vi "8_1_2.vi"() -> ()   [LabVIEW 2021, in "2022.lvlib"]
uses:
  2022.lvlib
panel:
  in  "8_1/2":bool=TRUE
  out "max value":i32
  out "size(s)":i32
  out "Array 2":bool[][](array[boolean])
  out "Array":i32[][](array[numeric])
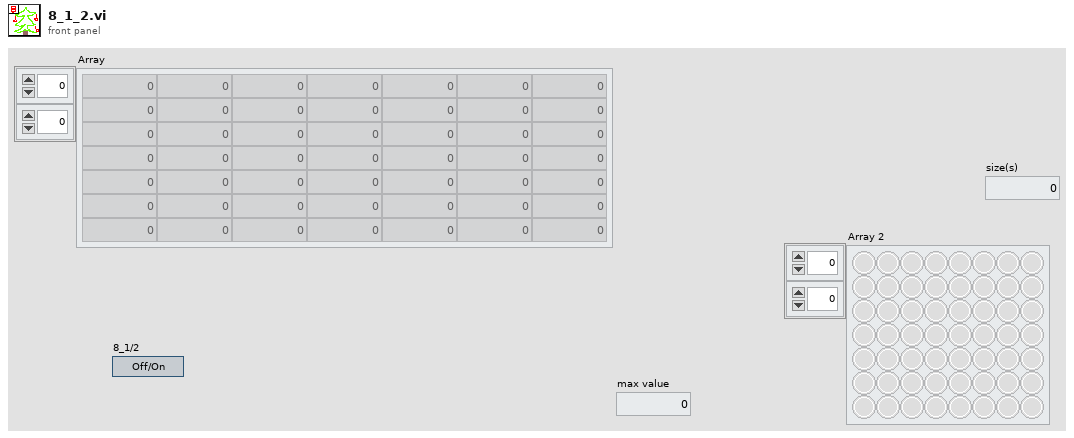
[diagram p1: front panel]
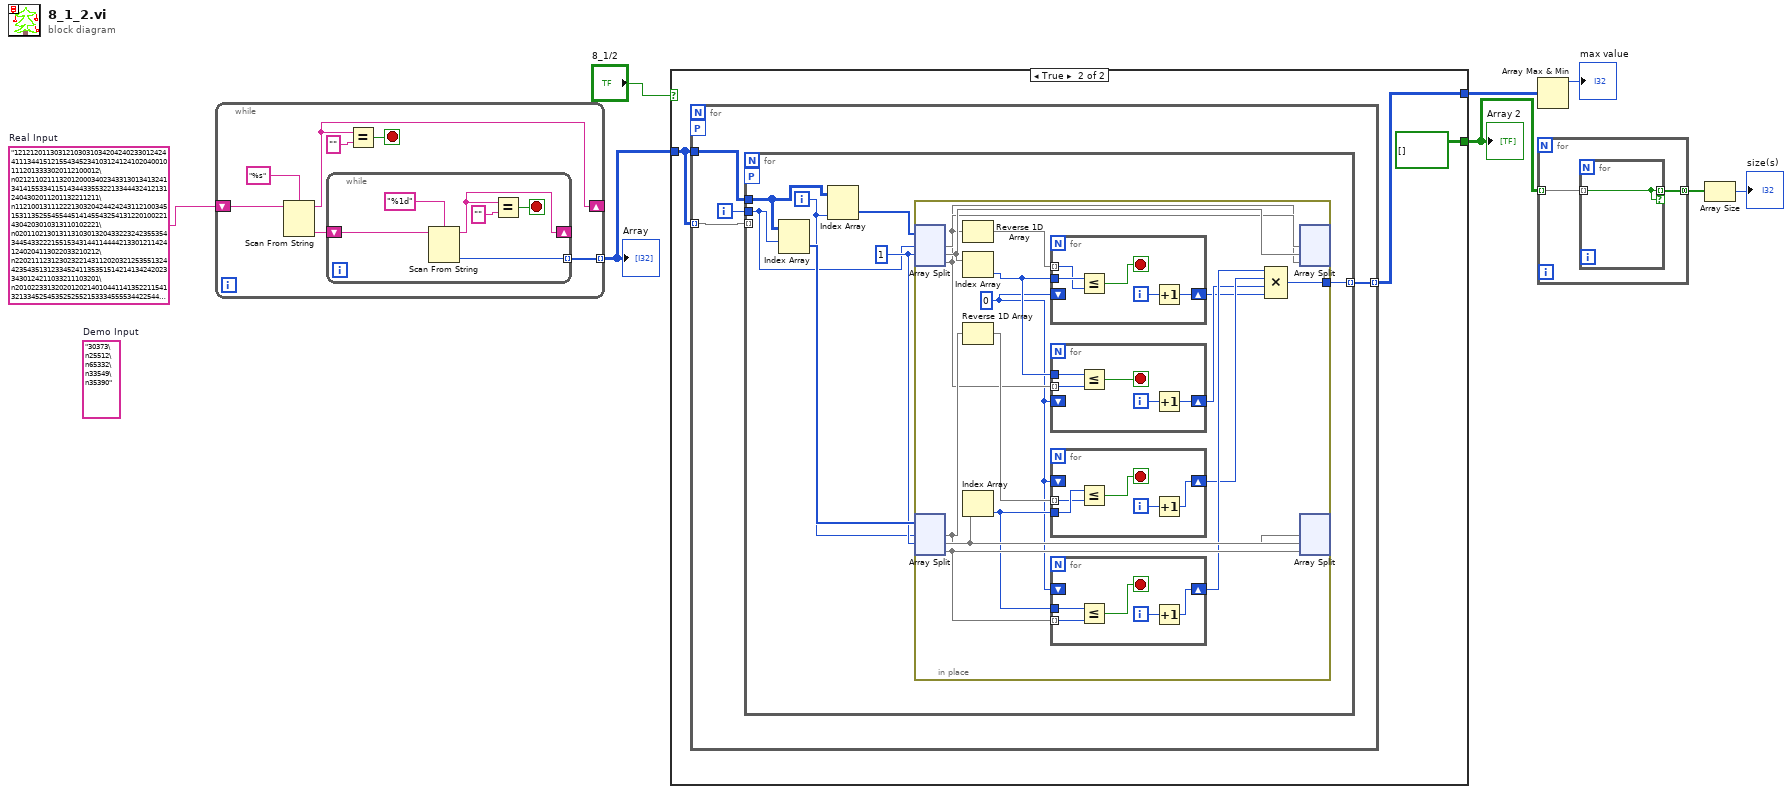
[diagram p0: block diagram]
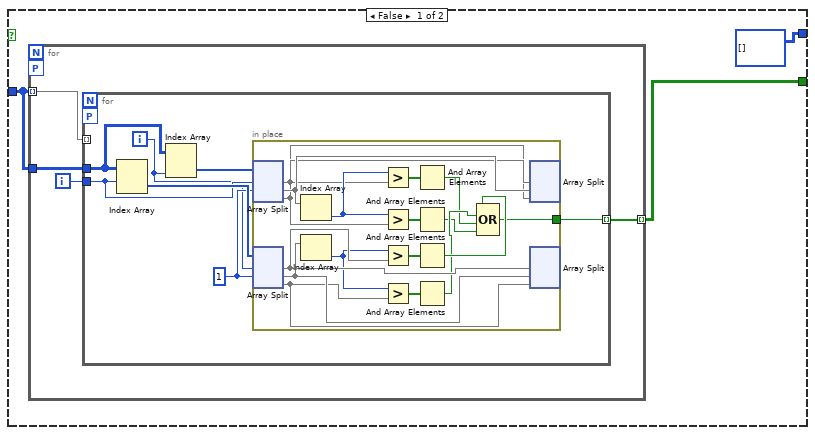
[diagram p2: hidden frame]
diagram:
  (unwired) "30373\n25512\n65332\n33549\n35390"  # Demo Input
  w3 = "121212011303121030310342042402330124244111344151215543452341031241241020400101112013333020112100012\n021211021113201200034023433130134132413414155334115143443355322133444324121312404302011201132211211\n112100131112221303204244242431121003451531135255455445141455432541312201002214304203010313110102221\n020110213013113103013204332232423553543445433222155153431441144442133012114241240204113022033210212\n220211123123023221431120203212535513244235435131233452411353515142141342420233430124211033211103201\n201022331320201202140104411413522115413213345254535252552153334555534422544330002102424023033322310\n..."  # Real Input
  n1 = while {
    shift-right: [w10] -> _
    shift-left: w3 -> [w15]
    tunnel: [w9] -> w8 mode=indexing
    stop <- w12 stop-if-true
    n2 = Scan From String(format string="%s", input string=w15) -> (remaining string=w10:string, output 1=w11:string)  [unwired: 3 in, 2 out]
    n3 = while {
      shift-right: [w19] -> _
      shift-left: w11 -> [w21]
      tunnel: [w17] -> w9 mode=indexing
      stop <- w16 stop-if-true
      n4 = Scan From String(format string="%1d", input string=w21) -> (remaining string=w19:string, output 1=w17:i32)  [unwired: 3 in, 2 out]
      n5 = Equal?(x=w19, y="") -> (x = y?=w16:bool)
    }
    n6 = Equal?(x=w10, y="") -> (x = y?=w12:bool)
  }
  "Array" <- w8
  n7 = case shown="True" "8_1/2" {
    tunnel: w8 -> [w24 w55]
    tunnel: [w23 bool[][] []] -> w7
    tunnel: [i32[][] [] w54] -> w2
    frame False {
      n8 = for {
        tunnel: w24 -> [w28] mode=indexing
        tunnel: w24 -> [w27]
        tunnel: [w25] -> w23 mode=indexing
        workers-P: _ -> [_]
        i -> [w26]
        n9 = for {
          tunnel: w28 -> [_] mode=indexing
          tunnel: w27 -> [w35]
          tunnel: w26 -> [w30]
          tunnel: [w31] -> w25 mode=indexing
          workers-P: _ -> [_]
          i -> [w29]
          w32 = 1
          n10 = Index Array(array=w35, index (row)=w30) -> (element=w34:i32[])  [unwired: 1 in]
          n11 = Index Array(array=w35, index (col)=w29) -> (element=w33:i32[])  [unwired: 1 in]
          n12 = in-place {
            in-place-border: [w36] -> w31
            n13 = in-place-split #1(w33, w30, w32) -> (w42:i32[], w51:i32[], w41:i32[])
            n14 = in-place-split #2(w34, w29, w32) -> (w49:i32[], w52:i32[], w47:i32[])
            n15 = Index Array(array=w51) -> (element=w43:i32)  [unwired: 1 in]
            n16 = Index Array(array=w52) -> (element=w48:i32)  [unwired: 1 in]
            n17 = Greater?(x=w43, y=w42) -> (0:w45:bool[])
            n18 = Greater?(x=w43, y=w41) -> (0:w44:bool[])
            n19 = Greater?(x=w48, y=w49) -> (0:w50:bool[])
            n20 = Greater?(x=w48, y=w47) -> (0:w46:bool[])
            n21 = And Array Elements(Boolean array=w45) -> (logical AND=w38:bool)
            n22 = And Array Elements(Boolean array=w44) -> (logical AND=w37:bool)
            n23 = And Array Elements(Boolean array=w50) -> (logical AND=w40:bool)
            n24 = And Array Elements(Boolean array=w46) -> (logical AND=w39:bool)
            n25 = Compound Arithmetic op=OR(w40, w39, w38, w37) -> (w36:bool)
            n26 = in-place-split #1(w42, w51, w41) -> ()  [unwired: 3 out]
            n27 = in-place-split #2(w49, w52, w47) -> ()  [unwired: 3 out]
          }
        }
      }
    }
    frame True {
      n28 = for {
        tunnel: w55 -> [w59] mode=indexing
        tunnel: w55 -> [w58]
        tunnel: [w56] -> w54 mode=indexing
        workers-P: _ -> [_]
        i -> [w57]
        n29 = for {
          tunnel: w59 -> [_] mode=indexing
          tunnel: w58 -> [w66]
          tunnel: w57 -> [w62]
          tunnel: [w60] -> w56 mode=indexing
          workers-P: _ -> [_]
          i -> [w61]
          w63 = 1
          n30 = Index Array(array=w66, index (row)=w62) -> (element=w65:i32[])  [unwired: 1 in]
          n31 = Index Array(array=w66, index (col)=w61) -> (element=w64:i32[])  [unwired: 1 in]
          n32 = in-place {
            in-place-border: [w80] -> w60
            w67 = 0
            n33 = in-place-split #3(w64, w62, w63) -> (w75:i32[], w81:i32[], w72:i32[])
            n34 = in-place-split #4(w65, w61, w63) -> (w78:i32[], w82:i32[], w79:i32[])
            n35 = Reverse 1D Array(array=w75) -> (reversed array=w74:i32[])
            n36 = Index Array(array=w81) -> (element=w73:i32)  [unwired: 1 in]
            n37 = Reverse 1D Array(array=w78) -> (reversed array=w77:i32[])
            n38 = Index Array(array=w82) -> (element=w76:i32)  [unwired: 1 in]
            n39 = for {
              tunnel: w73 -> [w87]
              tunnel: w74 -> [w86] mode=indexing
              shift-right: [w84] -> w68
              shift-left: w67 -> [_]
              i -> [w85]
              stop <- w83 stop-if-true
              n40 = Less Or Equal?(x=w87, y=w86) -> (x <= y?=w83:bool)
              n41 = Increment(x=w85) -> (x+1=w84:i32)
            }
            n42 = for {
              tunnel: w73 -> [w92]
              tunnel: w72 -> [w91] mode=indexing
              shift-right: [w89] -> w69
              shift-left: w67 -> [_]
              i -> [w90]
              stop <- w88 stop-if-true
              n43 = Less Or Equal?(x=w92, y=w91) -> (x <= y?=w88:bool)
              n44 = Increment(x=w90) -> (x+1=w89:i32)
            }
            n45 = for {
              tunnel: w76 -> [w97]
              tunnel: w77 -> [w96] mode=indexing
              shift-right: [w94] -> w70
              shift-left: w67 -> [_]
              i -> [w95]
              stop <- w93 stop-if-true
              n46 = Less Or Equal?(x=w97, y=w96) -> (x <= y?=w93:bool)
              n47 = Increment(x=w95) -> (x+1=w94:i32)
            }
            n48 = for {
              tunnel: w76 -> [w102]
              tunnel: w79 -> [w101] mode=indexing
              shift-right: [w99] -> w71
              shift-left: w67 -> [_]
              i -> [w100]
              stop <- w98 stop-if-true
              n49 = Less Or Equal?(x=w102, y=w101) -> (x <= y?=w98:bool)
              n50 = Increment(x=w100) -> (x+1=w99:i32)
            }
            n51 = Compound Arithmetic op=MULTIPLY(w71, w70, w69, w68) -> (w80:i32)
            n52 = in-place-split #3(w75, w81, w72) -> ()  [unwired: 3 out]
            n53 = in-place-split #4(w78, w82, w79) -> ()  [unwired: 3 out]
          }
        }
      }
    }
  }
  "Array 2" <- w7
  n54 = Array Max & Min(array=w2) -> (max value=→"max value":i32)  [unwired: 3 out]
  n55 = for {
    tunnel: w7 -> [w104] mode=indexing
    tunnel: [w103] -> w6 mode=concatenating
    n56 = for {
      tunnel: w104 -> [w105] mode=indexing
      tunnel: [w105] -> w103 mode=indexing if=w105
    }
  }
  n57 = Array Size(array=w6) -> (size(s)=→"size(s)":i32)
